vi "rethinkdb_msg_auth_client_final.vi"(8 "error in (no error)":errorcluster, 10 "client hash":u32[](array[numeric])=[3924058078, 3517073993, 456916219, 4181474074, 721615099, 493021554, 2954362323, 1579285327] format="%08x", 11 "auth server first":string="r=E9E45FDED1A24A491B3BFCFBF93C3B1A2B02F8FB1D62E972B017FDD35E21FB4F23qZziq9CEH0+7+F0ncN,s=mgBQZ0/scyBmiOLE7dFdKg==,i=4096") -> (0 "error out":errorcluster, 3 "auth client final":string)   [LabVIEW 2017]
panel:
  out "from base64":string
  out "server concate":string
  out "sha-256 hash":u32[](array[numeric]) format="%08x"
  out "client hash valid?":bool
  out "client hash 2":u32[](array[numeric]) format="%08x"
  out "msg":T1
  out "r":string
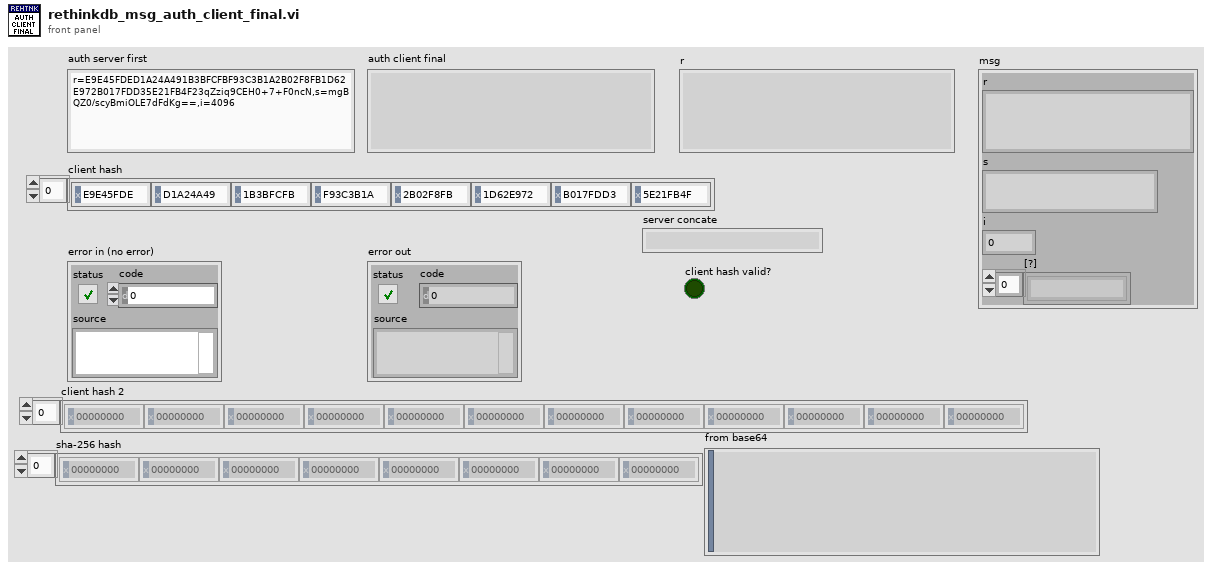
[diagram p1: front panel]
types:
  T1 = cluster{"r":string, "s":string, "i":i32, "[?]":string[]}
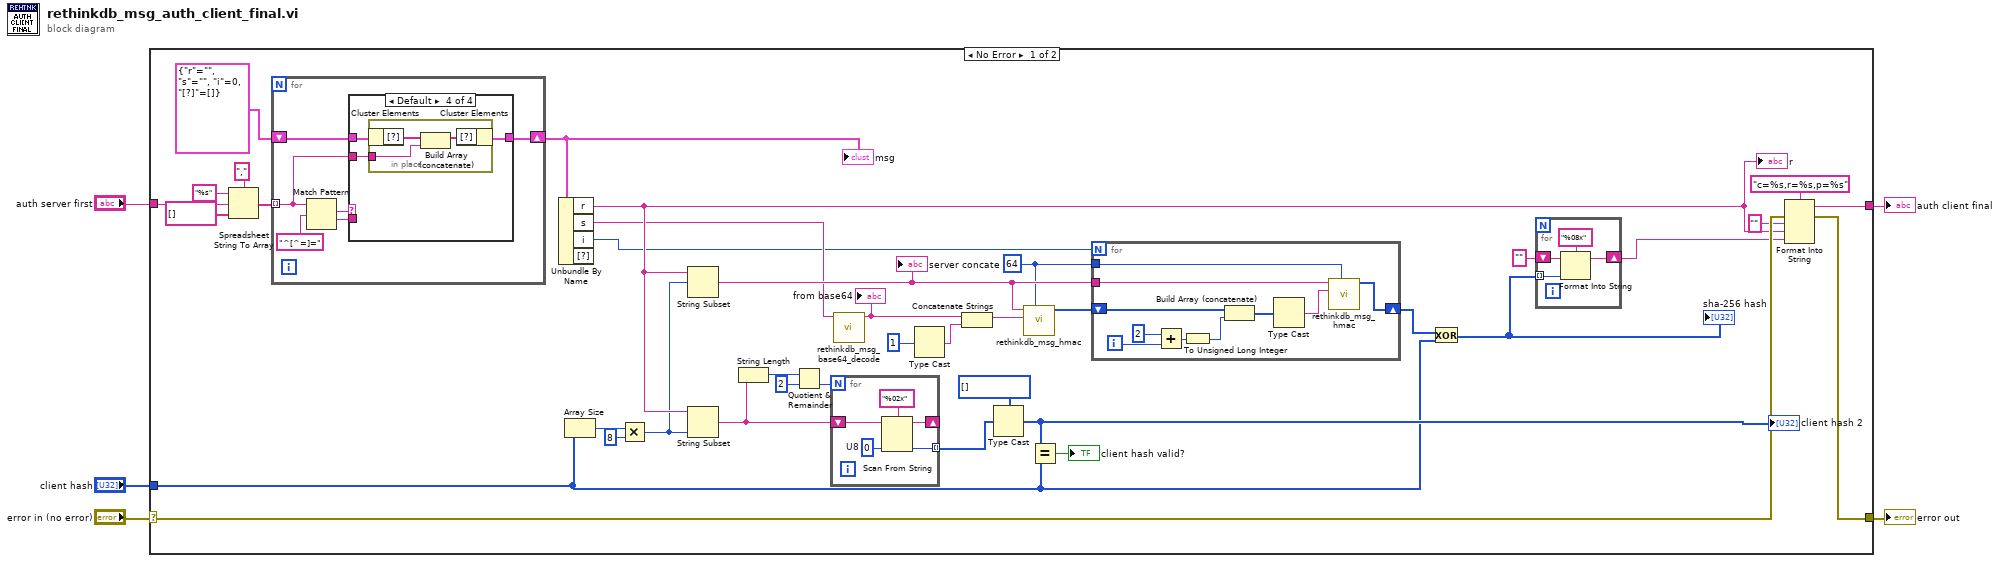
[diagram p0: block diagram]
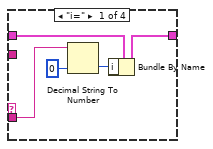
[diagram p2: hidden frame]
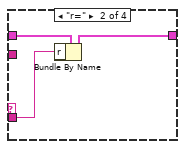
[diagram p3: hidden frame]
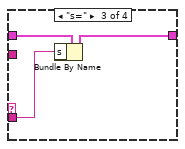
[diagram p4: hidden frame]
diagram:
  n1 = case shown="No Error" "error in (no error)" {
    selector: "error in (no error)" -> [w37 w86]
    tunnel: [w36 w86] -> w4
    tunnel: [w35 _] -> w3
    tunnel: "auth server first" -> [w43 _]
    tunnel: "client hash" -> [w9 _]
    frame No Error {
      w17 = 64 ("blocksize (SHA256=64)")
      n2 = Spreadsheet String To Array(delimiter (Tab)=",", format string="%s", spreadsheet string=w43, array type (2D Dbl)=string[] []) -> (array=w39:string[])
      n3 = for {
        tunnel: w39 -> [w63] mode=indexing
        shift-right: [w65] -> w32
        shift-left: T1 {"r"="", "s"="", "i"=0, "[?]"=[]} ("msg") -> [w64]
        n4 = Match Pattern(string=w63, regular expression="^[^=]=") -> (match substring=w67:string, after substring=w66:string)  [unwired: 1 in, 2 out]
        n5 = case shown="Default" w67 {
          tunnel: w66 -> [w71 w74 w77 _]
          tunnel: [w72 w75 w78 w80] -> w65
          tunnel: w64 -> [w73 w76 w79 w82]
          tunnel: w63 -> [_ _ _ w81]
          frame "i=" {
            n6 = Decimal String To Number(string=w71, default (0L)=0 ("default (0 I32)")) -> (number=w70:i32)  [unwired: 1 in, 1 out]
            n7 = Bundle By Name(cluster=w73, "i"=w70) -> (w72:T1)
          }
          frame "r=" {
            n8 = Bundle By Name(cluster=w76, "r"=w74) -> (w75:T1)
          }
          frame "s=" {
            n9 = Bundle By Name(cluster=w79, "s"=w77) -> (w78:T1)
          }
          frame Default {
            n10 = in-place {
              in-place-border: w81 -> [w83]
              n11 = in-place-cluster #1(w82) -> ("[?]"=w85:string[])
              n12 = Build Array (concatenate)(w85, w83) -> (w84:string[])
              n13 = in-place-cluster #1("[?]"=w84) -> (w80:T1)
            }
          }
        }
      }
      "msg" <- w32
      n14 = Unbundle By Name(w32) -> ("r"=w21:string, "s"=w16:string, "i"=w13:i32)  [unwired: 1 out]
      "r" <- w21
      n15 = Array Size(array=w9) -> (size(s)=w26:i32)
      n16 = Multiply(x=w26, y=8) -> (x*y=w20:i32)
      n17 = String Subset(string=w21, offset (0)=w20) -> (substring=w19:string)  [unwired: 1 in]
      "server concate" <- w19
      n18 = String Subset(string=w21, length (rest)=w20) -> (substring=w24:string)  [unwired: 1 in]
      n19 = String Length(string=w24) -> (length=w28:i32)
      n20 = Quotient & Remainder(x=w28, y=2) -> (floor(x/y)=w29:i32)  [unwired: 1 out]
      n21 = for {
        N: w29 -> [_]
        shift-right: [w59] -> _
        shift-left: w24 -> [w60]
        tunnel: [w58] -> w31 mode=indexing
        w61 = u8 0  # U8
        n22 = Scan From String(format string="%02x", input string=w60, default 1=w61) -> (remaining string=w59:string, output 1=w58:u8)  [unwired: 2 in, 2 out]
      }
      n23 = call "rethinkdb_msg_base64_decode.vi"("base64"=w16) -> ("string"=w15:string)  [unwired: 10 in]
      "from base64" <- w15
      n24 = Type Cast(x=1) -> (*(type *) &x=w12:string)  [unwired: 1 in]
      n25 = Concatenate Strings(w15, w12) -> (w11:string)
      n26 = Type Cast(type=u32[] [], x=w31) -> (*(type *) &x=w23:u32[])
      "client hash 2" <- w23
      n27 = call "rethinkdb_msg_hmac.vi"("blocksize (SHA256=64)"=w17, "message"=w11, "key"=w19) -> ("sha-256 hash"=w18:u32[])  [unwired: 8 in]
      n28 = Equal?(x=w23, y=w9) -> (x = y?=→"client hash valid?":bool)
      n29 = for {
        N: w13 -> [_]
        tunnel: w19 -> [w57]
        tunnel: w17 -> [w56]
        shift-right: [w55] -> w10
        shift-left: w18 -> [w52]
        i -> [w54]
        n30 = Add(x=2, y=w54) -> (x+y=w51:i32)
        n31 = To Unsigned Long Integer(number=w51) -> (unsigned 32bit integer=w50:u32)
        n32 = Build Array (concatenate)(w52, w50) -> (w49:u32[])
        n33 = Type Cast(x=w49) -> (*(type *) &x=w48:string)  [unwired: 1 in]
        n34 = call "rethinkdb_msg_hmac.vi"("blocksize (SHA256=64)"=w56, "message"=w48, "key"=w57) -> ("sha-256 hash"=w55:u32[])  [unwired: 8 in]
      }
      n35 = Exclusive Or(1:w9, 2:w10) -> (0:w7:u32[])
      "sha-256 hash" <- w7
      n36 = for {
        tunnel: w7 -> [w46] mode=indexing
        shift-right: [w45] -> w6
        shift-left: "" -> [w44]
        n37 = Format Into String(format string="%08x", initial string=w44, w46) -> (resulting string=w45:string)  [unwired: 1 in, 1 out]
      }
      n38 = Format Into String(format string="c=%s,r=%s,p=%s", error in=w37, "" ("input 1"), w21, w6) -> (resulting string=w35:string, error out=w36:errorcluster)  [unwired: 1 in]
    }
    frame Error {
    }
  }
  "error out" <- w4
  "auth client final" <- w3
